vi "Continuous Sampling Arduino.vi"() -> ()   [LabVIEW 2014]
uses:
  <vilib>/express/express analysis/Spectral/Block/exnSpectralBlock spectral measurements PSD poly.vi
  <vilib>/express/express analysis/Spectral/Block/exnSpectralBlock spectral measurements PSD DDT.vi
  <vilib>/express/express analysis/Spectral/XNode/ExpressSpectralMeasurementsBlockNode.xnode
  <vilib>/LabVIEW Interface for Arduino/LabVIEW Interface for Arduino.lvlib
panel:
  out "Executiontime per Loop":u32
  in  "Sample Rate (HZ)":u16=5000
  in  "Analog Input Pin":u8
  in  "Stop":bool
  out "Waveform Chart":waveform(dbl)(graph)
  in  "Lower Cut-Off":dbl=100.0 min=0.0 max=2499.0 step=10.0
  out "Processed Chart":dynamicdata(graph)
  out "Spectrum":dynamicdata(graph)
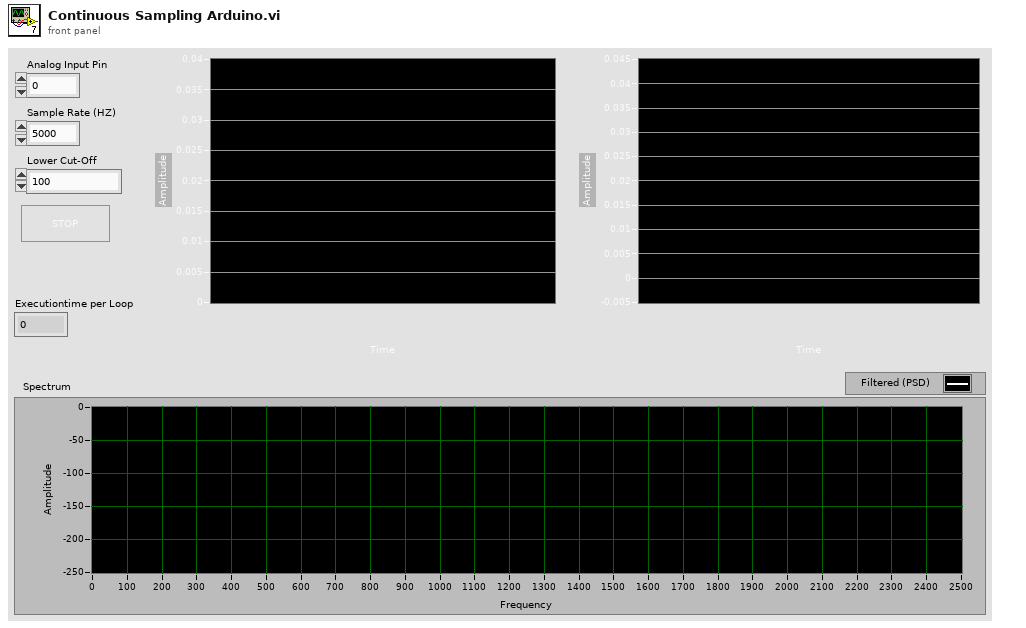
[diagram p1: front panel]
types:
  T1 = typedef "LabVIEW Interface for Arduino.lvlib/Arduino Resource.ctl" = cluster{"VISA resource":refnum<visa-resource-name>, "Board Type":T2, "Connection Type":enum8{"USB / Serial"}, "Bytes Per Packet (15)":u8}
  T2 = typedef "LabVIEW Interface for Arduino.lvlib/Board Type.ctl" = enum16{"Uno", "Dimuelanove w/Atmega 328", "Mega 2560"}
  T3 = cluster{"averaging mode":u16, "weighting mode":u16, "number of averages":u32}
  T4 = cluster{"dB On (F)":bool, "unwrap phase (F)":bool, "convert to degree (F)":bool}
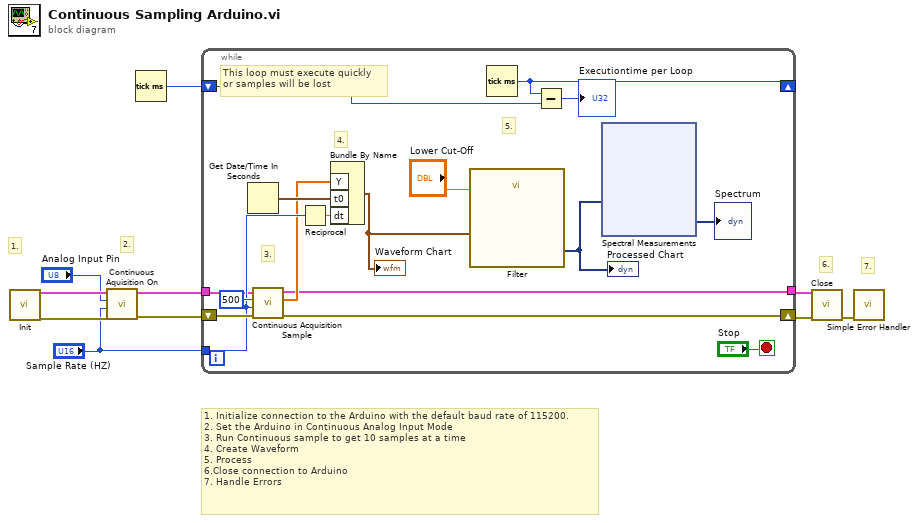
[diagram p0: block diagram]
diagram:
  # "7."
  # "6."
  # "2."
  # "1."
  # "1. Initialize connection to the Arduino with the default baud rate of 115200.\n2. Set the Arduino in Continuous Analog Input Mode\n3. Run Continuous sample to get 10 samples at a time\n4. Create Waveform \n5. Process\n6.Close connection to Arduino\n7. Handle Errors"
  n1 = call <vilib>:"Init.vi"() -> ("Arduino Resource"=w10:T1, "error out"=w5:errorcluster)  [unwired: 18 in]
  n2 = call <vilib>:"Continuous Aquisition On.vi"("error in"=w5, "Acquition Speed"="Sample Rate (HZ)", "Analog Input Pin"="Analog Input Pin", "Arduino Resource"=w10) -> ("error out"=w2:errorcluster, "Arduino Resource"=w3:T1)  [unwired: 6 in]
  n3 = Tick Count (ms)() -> (millisecond timer value=w1:u32)
  n4 = while {
    tunnel: [w17] -> w9
    shift-right: [w16] -> w6
    shift-left: w2 -> [w26]
    tunnel: "Sample Rate (HZ)" -> [w21]
    tunnel: w3 -> [w14]
    shift-right: [w12] -> _
    shift-left: w1 -> [w13]
    stop <- "Stop" stop-if-true
    # "5."
    # "4."
    # "This loop must execute quickly\nor samples will be lost"
    # "3."
    n5 = Get Date/Time In Seconds() -> (seconds since 1Jan1904=w20:timestamp)
    n6 = call <vilib>:"Continuous Acquisition Sample.vi"("Arduino Resource"=w14, "Samples to Read"=u16 500, "Sample Rate (HZ)"=w21, "error in (no error)"=w26) -> ("Arduino Resource"=w17:T1, "Data"=w19:dbl[], "error out"=w16:errorcluster)  [unwired: 4 in]
    n7 = Reciprocal(x=w21) -> (1/x=w22:dbl)
    n8 = Bundle By Name("Y"=w19, "t0"=w20, "dt"=w22) -> (w18:waveform(dbl))  [unwired: 1 in]
    "Waveform Chart" <- w18
    n9 = call "Filter"("Lower Cut-Off"="Lower Cut-Off", "Signal"=w18) -> ("Filtered Signal"=w15:dynamicdata)  [unwired: 8 in, 1 out]
    "Processed Chart" <- w15
    n10 = Tick Count (ms)() -> (millisecond timer value=w12:u32)
    n11 = Subtract(x=w12, y=w13) -> (x-y=→"Executiontime per Loop":u32)
    n12 = xnode "Spectral Measurements"("Signals"=w15) -> ("PSD"=→"Spectrum":dynamicdata)  [unwired: 1 in, 1 out]
  }
  n13 = call <vilib>:"Close.vi"("Arduino Resource"=w9, "error in"=w6) -> ("error out"=w8:errorcluster)  [unwired: 13 in]
  n14 = call <vilib>:"Simple Error Handler.vi"("error in (no error)"=w8) -> ()  [unwired: 4 in, 5 out]
